vi "Load All Subitems.vi"(8 "error in (no error)":errorcluster, 11 "Application Data in":T1) -> (0 "error out":errorcluster, 3 "Application Data out":T1)   [LabVIEW 2017, in "DSF Core.lvlib"]
uses:
  DSF Core.lvlib
  Main VI/Application Data.ctl
  <vilib>/NI/Memory Manager/Classes/Pointer/Pointer.lvclass
  Classes/Framework/Framework.lvclass
  Buffer Reader/Buffer Data.ctl
  Classes/Buffer/Buffer.lvclass
  Classes/Transfer Group Status/Transfer Group Status.lvclass
  Classes/Framework/Framework.lvclass/Framework.ctl
  Classes/Plugin/Plugin.lvclass/Plugin.ctl
  Classes/Timing/Timing.lvclass/Timing.ctl
  Classes/Transfer Group/Transfer Group.lvclass/Transfer Group.ctl
  Classes/Transfer/Transfer.lvclass/Transfer.ctl
  Classes/Buffers/Buffers.lvclass/Buffers.ctl
  Add Plugin with Children.vi
  Classes/Framework/Get Async Plugins.vi
  Classes/Framework/Get Inline Plugins.vi
  Classes/Plugin/Get Name.vi
  Create New Tree Item.vi
  Add Transfer Group with Children.vi
  Classes/Plugin/Get Inline Tx Transfer Groups.vi
  Classes/Plugin/Get Async Rx Transfer Groups.vi
  Classes/Plugin/Get Async Tx Transfer Groups.vi
  Classes/Plugin/Get Inline Rx Transfer Groups.vi
  Add Buffer Data to Variant.vi
  Classes/Plugin/Get Timing.vi
  Classes/Timing/Get Decimation.vi
  Classes/Plugin/Get Buffers.vi
  Classes/Buffers/Get String Buffer.vi
  Classes/Transfer Group/Get Name.vi
  Add Transfer.vi
  Classes/Transfer Group/Get Transfers.vi
  Classes/Transfer Group/Get Inline.vi
  Classes/Transfer Group/Get Timing.vi
  Classes/Transfer Group/Get Status.vi
  Classes/Transfer/Get Name.vi
  Classes/Transfer/Get Buffers.vi
  Add Buffers.vi
  Classes/Buffers/Get Async Buffer.vi
  Classes/Buffers/Get Inline Buffer.vi
  Add Item to Tree.vi
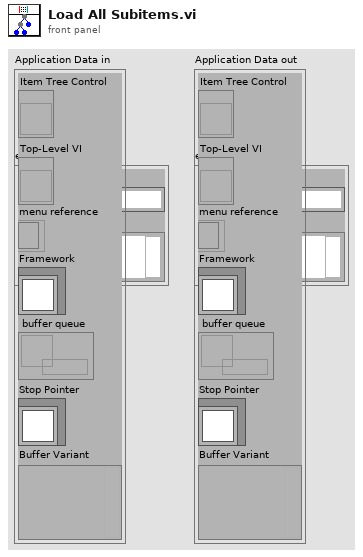
[diagram p1: front panel]
types:
  T1 = typedef "DSF Core.lvlib/Application Data.ctl" = cluster{"Item Tree Control":refnum<vi>, "Top-Level VI":refnum<vi>, "menu reference":refnum<k9>, "Framework":refnum<class "Framework.lvclass">, "buffer queue":refnum<queue>, "Stop Pointer":refnum<class "Pointer.lvclass">, "Buffer Variant":variant}
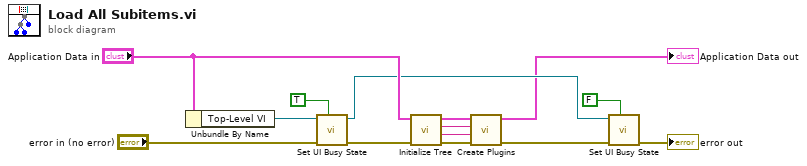
[diagram p0: block diagram]
diagram:
  n1 = Unbundle By Name("Application Data in") -> ("Top-Level VI"=w13:refnum<vi>)
  n2 = call "Set UI Busy State.vi"("Defer Panel Updates"=TRUE, "error in (no error)"="error in (no error)", "VI in"=w13) -> ("error out"=w8:errorcluster, "VI out"=w7:refnum<vi>)  [unwired: 7 in]
  n3 = call "Initialize Tree.vi"("error in (no error)"=w8, "Application Data in"="Application Data in") -> ("error out"=w6:errorcluster, "async plugins tag"=w1:string, "inline plugins tag"=w2:string, "Application Data out"=w5:T1)  [unwired: 6 in]
  n4 = call "Create Plugins.vi"("error in (no error)"=w6, "async plugins tag"=w1, "inline plugins tag"=w2, "Application Data In"=w5) -> ("error out"=w4:errorcluster, "Application Data out"=→"Application Data out":T1)  [unwired: 6 in]
  n5 = call "Set UI Busy State.vi"("Defer Panel Updates"=FALSE, "error in (no error)"=w4, "VI in"=w7) -> ("error out"=→"error out":errorcluster)  [unwired: 7 in, 1 out]
